vi "Stop Monitor.vi"(6 "Write to FPGA(T)":bool=TRUE, 8 "error in (no error)":errorcluster, 11 "FPGA VI Reference In":refnum<k20>) -> (0 "error out":errorcluster, 3 "FPGA VI Reference Out":refnum<k20>)   [LabVIEW 2016]
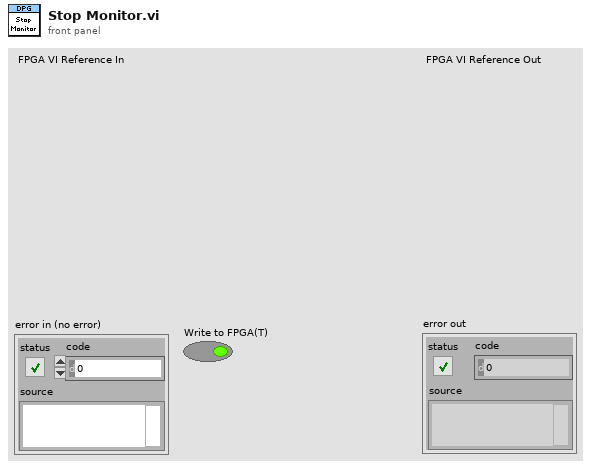
[diagram p1: front panel]
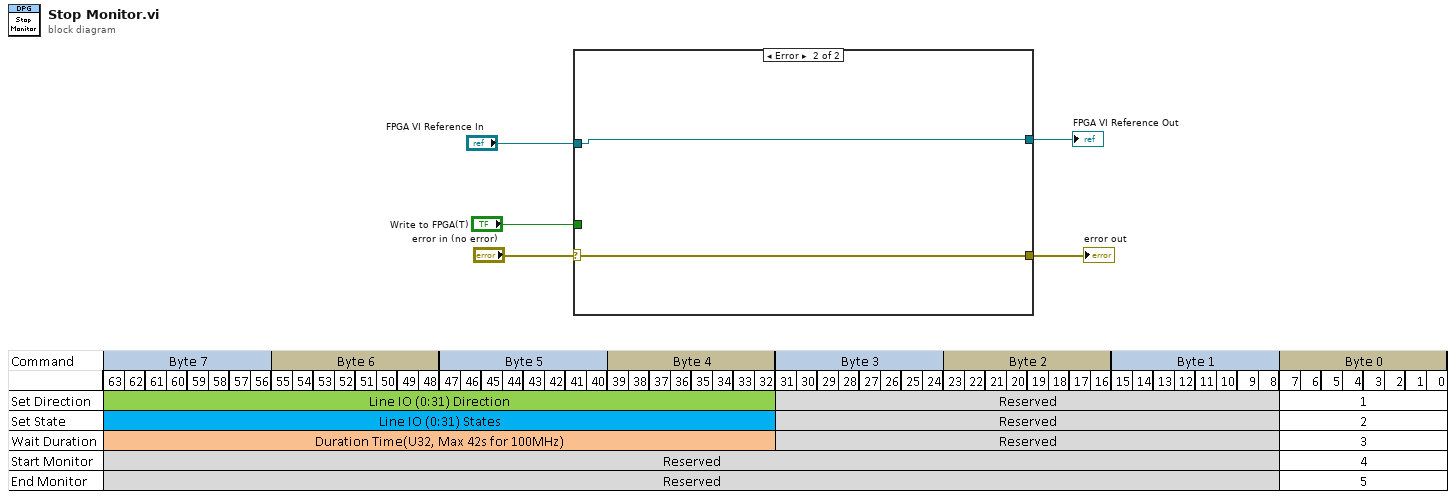
[diagram p0: block diagram]
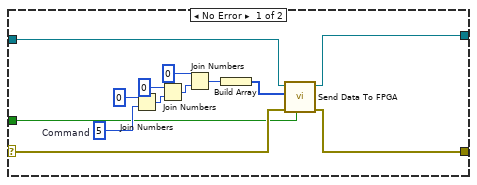
[diagram p2: hidden frame]
diagram:
  n1 = case shown="Error" "error in (no error)" {
    selector: "error in (no error)" -> [w10 w20]
    tunnel: "FPGA VI Reference In" -> [w13 w19]
    tunnel: [w8 w20] -> w3
    tunnel: "Write to FPGA(T)" -> [w9 _]
    tunnel: [w6 w19] -> w1
    frame No Error {
      w16 = u16 5  # Command
      n2 = Join Numbers(hi=u16 0, lo=w16) -> ((hi.lo)=w17:u32)
      n3 = Join Numbers(hi=u32 0, lo=w17) -> ((hi.lo)=w18:u64)
      n4 = Join Numbers(hi=u64 0, lo=w18) -> ((hi.lo)=w12:u64)
      n5 = Build Array(w12) -> (w11:u64[])
      n6 = call "Send Data To FPGA.vi"("Write to FPGA(T)"=w9, "error in (no error)"=w10, "Data"=w11, "FPGA VI Reference In"=w13) -> ("error out"=w8:errorcluster, "FPGA VI Reference Out"=w6:refnum<k20>)  [unwired: 6 in]
    }
    frame Error {
    }
  }
  "error out" <- w3
  "FPGA VI Reference Out" <- w1
